vi "DSP_ReadRAM.vi"(3 "error in (no error)":errorcluster, 4 "Samples To Read":u16, 5 "Board Handle":u64) -> (0 "error out":errorcluster, 1 "Values Out":u16[](array[numeric]), 2 "Board Handle Out":u64)   [LabVIEW 2009]
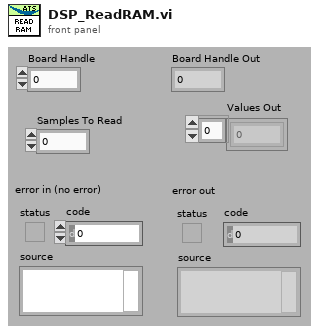
[diagram p1: front panel]
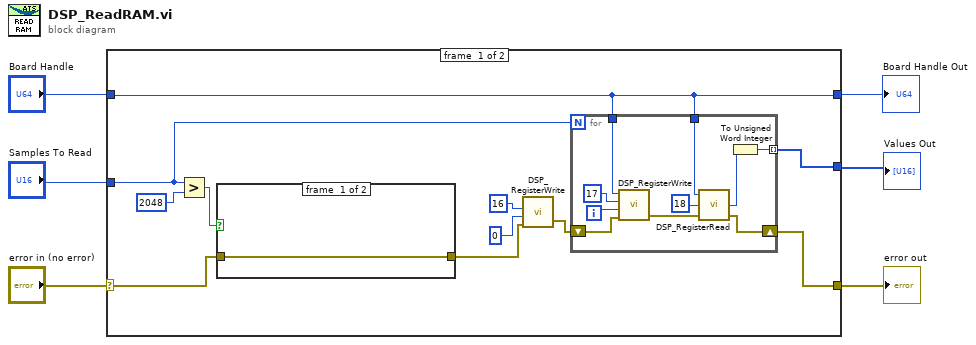
[diagram p0: block diagram]
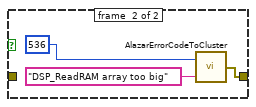
[diagram p2: hidden frame]
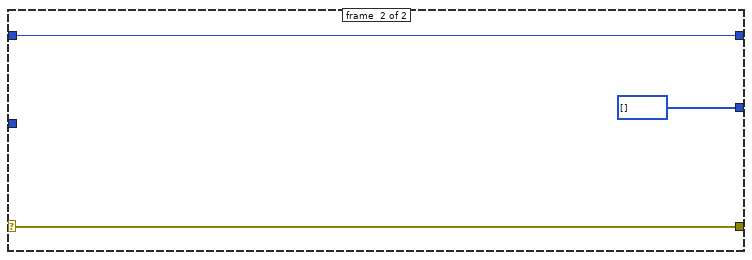
[diagram p3: hidden frame]
diagram:
  n1 = case shown="No Error" "error in (no error)" {
    selector: "error in (no error)" -> [w15 w34]
    tunnel: [w9 w34] -> w5
    tunnel: [w10 w33] -> w4
    tunnel: "Board Handle" -> [w10 w33]
    tunnel: [w8 u16[] []] -> w2
    tunnel: "Samples To Read" -> [w7 _]
    frame #0 {
      n2 = Greater?(x=w7, y=2048) -> (0:w16:bool)
      n3 = case shown="True" w16 {
        tunnel: w15 -> [w28 _]
        tunnel: [w28 w29] -> w11
        frame #0 {
        }
        frame #1 {
          n4 = call "AlazarErrorCodeToCluster.vi"("Message"="DSP_ReadRAM array too big", "Error Code"=u32 536) -> ("error out"=w29:errorcluster)
        }
      }
      n5 = call "DSP_RegisterWrite.vi"("error in (no error)"=w11, "Value"=u32 0, "Offset"=u32 16) -> ("error out"=w13:errorcluster)  [unwired: 1 in, 1 out]
      n6 = for {
        N: w7 -> [_]
        tunnel: w10 -> [w25]
        shift-right: [w20] -> w9
        shift-left: w13 -> [w24]
        tunnel: w10 -> [w23]
        tunnel: [w18] -> w8 mode=indexing
        i -> [w27]
        n7 = call "DSP_RegisterWrite.vi"("error in (no error)"=w24, "Value"=w27, "Offset"=u32 17, "Board Handle"=w25) -> ("error out"=w22:errorcluster)  [unwired: 1 out]
        n8 = call "DSP_RegisterRead.vi"("error in (no error)"=w22, "Offset"=u32 18, "Board Handle"=w23) -> ("error out"=w20:errorcluster, "Value"=w19:u32)  [unwired: 1 out]
        n9 = To Unsigned Word Integer(number=w19) -> (unsigned 16bit integer=w18:u16)
      }
    }
    frame #1 {
    }
  }
  "Board Handle Out" <- w4
  "error out" <- w5
  "Values Out" <- w2
